vi "Start Vision.vi"() -> ()   [LabVIEW 2015]
uses:
  <vilib>/vision/driver/NI_Vision_Acquisition_Software.lvlib
  <vilib>/userdefined/High Color/IMAQdx.ctl
  <resource>/objmgr/imaqdx.rc
  Vision info.vi
panel:
  in  "no":i32
  in  "yes":i32
  out "Image 2":T1(plugin-control)
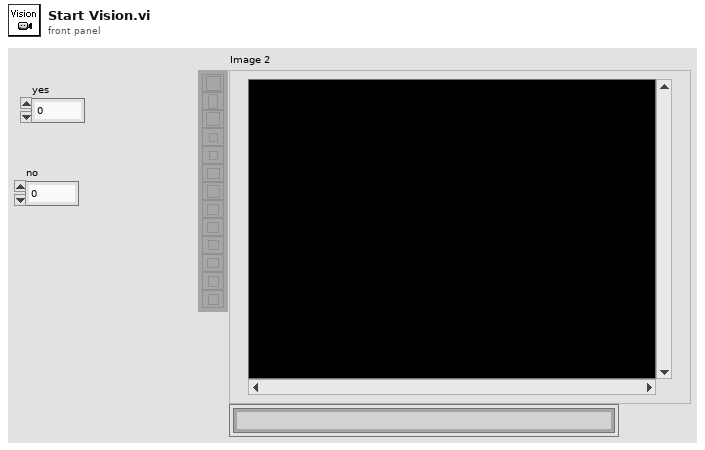
[diagram p1: front panel]
types:
  T1 = typedef "IMAQ Image.ctl" = refnum<image>
  T2 = typedef "IMAQdx.ctl" = refnum<k21>
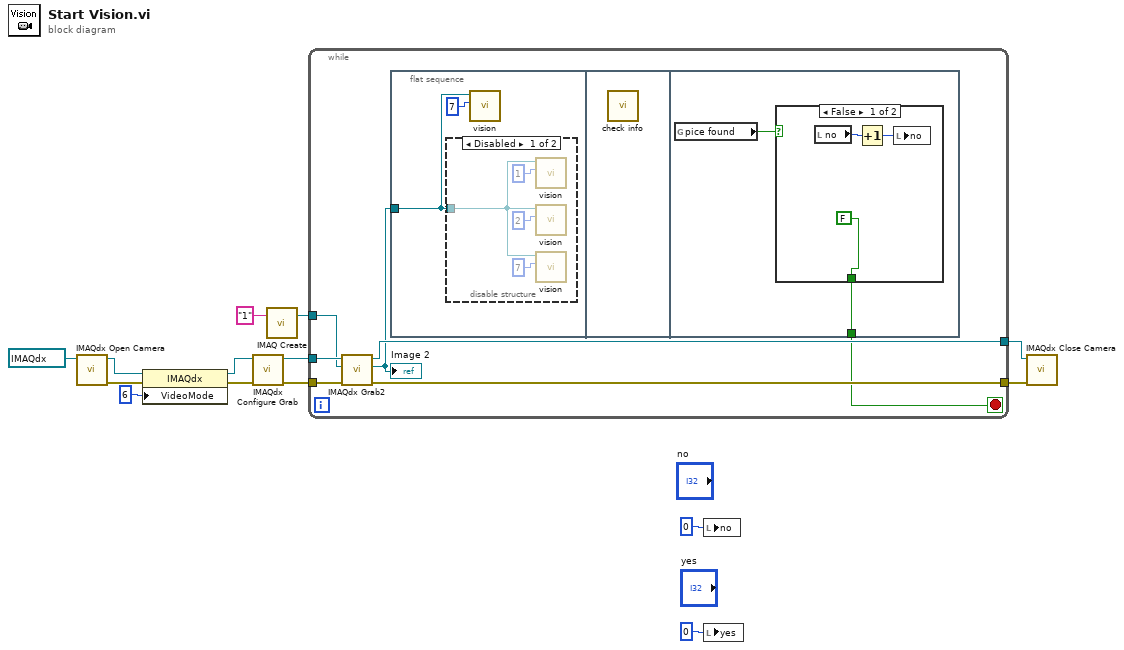
[diagram p0: block diagram]
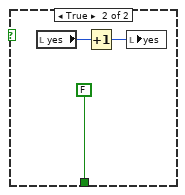
[diagram p3: hidden frame]
diagram:
  n1 = call <vilib>:"IMAQdx Open Camera.vi"("Session In"=T2 "cam0") -> ("error out"=w6:errorcluster, "Session Out"=w7:T2)  [unwired: 9 in]
  n2 = property class="IMAQdx"(reference=w7, error in=w6, "VideoMode"=u32 6) -> (reference out=w4:T2, error out=w5:errorcluster)
  n3 = call <vilib>:"IMAQdx Configure Grab.vi"("error in"=w5, "Session In"=w4) -> ("error out"=w13:errorcluster, "Session Out"=w12:T2)  [unwired: 8 in]
  n4 = call "IMAQ Create"("Image Name"="1") -> ("New Image"=w10:T1)  [unwired: 4 in, 1 out]
  n5 = while {
    tunnel: w13 -> [w21]
    tunnel: w12 -> [w20]
    tunnel: [w19] -> w11
    tunnel: w10 -> [w18]
    tunnel: [w17] -> w8
    stop <- w15 stop-if-true
    n6 = call <vilib>:"IMAQdx Grab2.vi"("error in"=w21, "Image In"=w18, "Session In"=w20) -> ("error out"=w17:errorcluster, "Image Out"=w16:T1, "Session Out"=w19:T2)  [unwired: 5 in, 1 out]
    "Image 2" <- w16
    n7 = flat-sequence {
      tunnel: w16 -> [w22]
      tunnel: [w28] -> w15
      frame #0 {
        n8 = disable-structure shown="Disabled" {
          disable-tunnel: w22 -> [w24 _]
          frame Disabled {
            n9 = call "vision.vi"("Color Plane"=1, "Refnum in"=w24) -> ()  [unwired: 10 in]
            n10 = call "vision.vi"("Color Plane"=2, "Refnum in"=w24) -> ()  [unwired: 10 in]
            n11 = call "vision.vi"("Color Plane"=7, "Refnum in"=w24) -> ()  [unwired: 10 in]
          }
          frame Enabled {
          }
        }
        n12 = call "vision.vi"("Color Plane"=7, "Refnum in"=w22) -> ()  [unwired: 10 in]
      }
      frame #1 {
        n13 = call "check info.vi"() -> ()  [unwired: 12 in]
      }
      frame #2 {
        n14 = global read "Vision info.vi" "pice found"() -> (w29:bool)
        n15 = case shown="False" w29 {
          tunnel: [FALSE FALSE] -> w28
          frame False {
            n16 = local read "no"() -> (w31:i32)
            n17 = Increment(x=w31) -> (x+1=w32:i32)
            n18 = local write "no"(w32) -> ()
          }
          frame True {
            n19 = local read "yes"() -> (w34:i32)
            n20 = Increment(x=w34) -> (x+1=w35:i32)
            n21 = local write "yes"(w35) -> ()
          }
        }
      }
    }
  }
  n22 = local write "no"(0 ("no")) -> ()
  n23 = local write "yes"(0 ("yes")) -> ()
  n24 = call <vilib>:"IMAQdx Close Camera.vi"("error in"=w8, "Session In"=w11) -> ()  [unwired: 9 in, 1 out]
